vi "Ib.vi"(0 "Case":enum16{"100uA", "200uA", "300uA"}(ring), 1 "Zasilacz BM572":refnum<visa-resource-name>) -> (2 "COMMAND":string)   [LabVIEW 2023]
doc: "Podajemy prad bazy i ustawiamy napicie na zasilaczu zgodne z danym prdem"
uses:
  Open_device_2018.llb/Select_Instr.ctl
panel:
  out "result string":string
  out "ERROR\nERROR":errorcluster
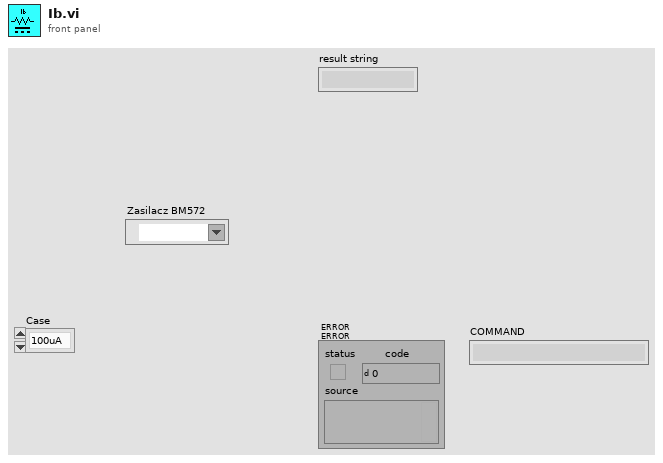
[diagram p1: front panel]
types:
  T1 = typedef "Select_Instr.ctl" = string
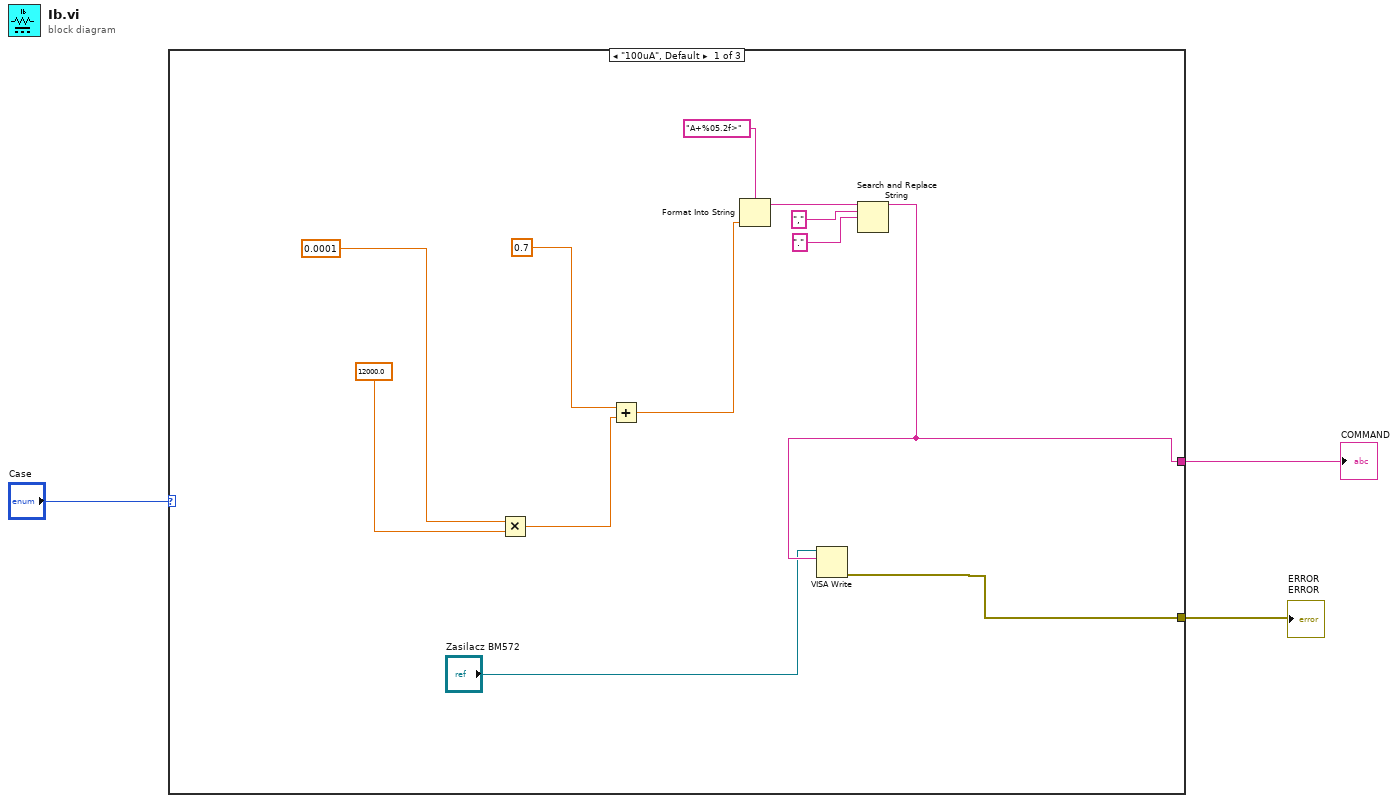
[diagram p0: block diagram]
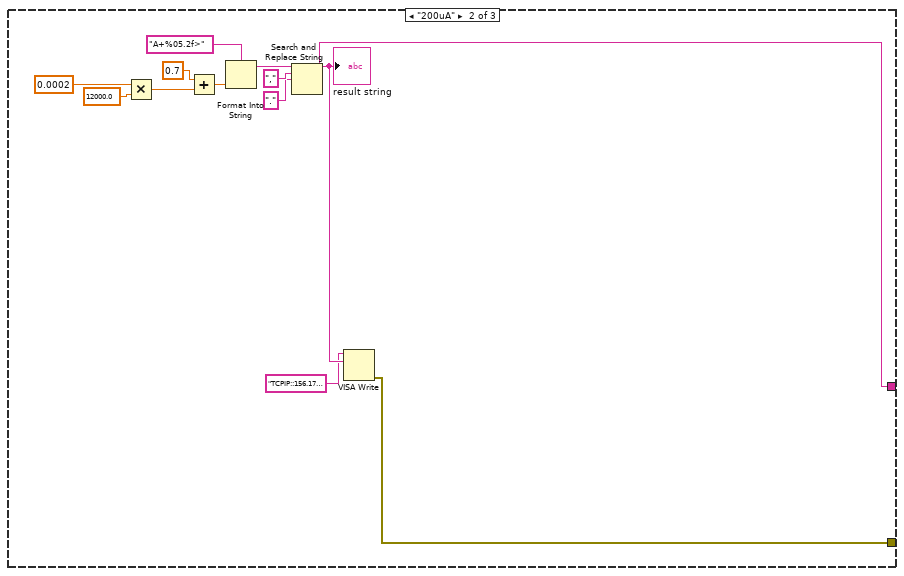
[diagram p2: hidden frame]
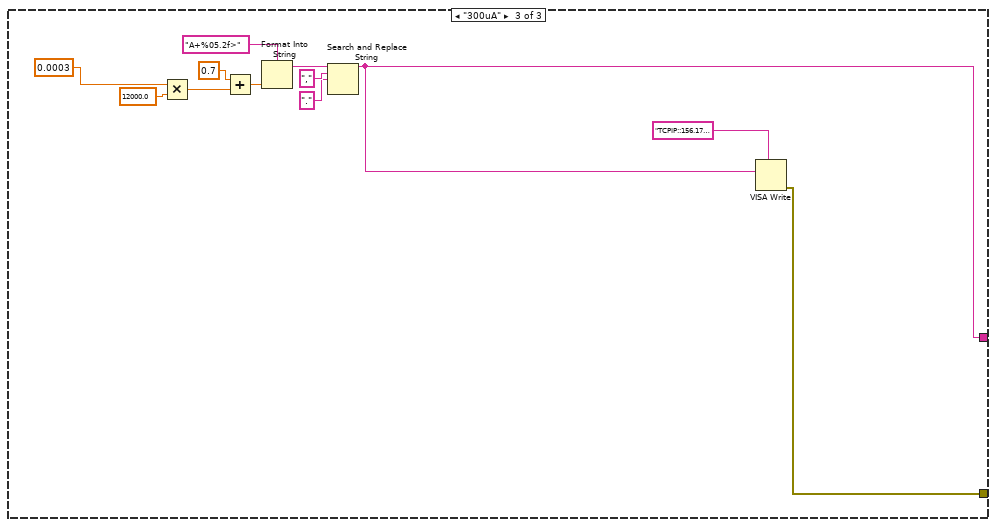
[diagram p3: hidden frame]
diagram:
  n1 = case shown="\"100uA\", Default" "Case" {
    tunnel: [w6 w18 w29] -> w3
    tunnel: [w7 w19 w31] -> w2
    frame "100uA", Default {
      n2 = Multiply(x=0.0001 ("Ib [A]"), y=12000.0) -> (x*y=w13:dbl)
      n3 = Add(x=0.7, y=w13) -> (x+y=w14:dbl)
      n4 = Format Into String(format string="A+%05.2f>" ("initial string"), w14) -> (resulting string=w15:string)  [unwired: 2 in, 1 out]
      n5 = Search and Replace String(input string=w15, search string=",", replace string="." ("replace string (\"\")")) -> (result string=w7:string)  [unwired: 5 in, 3 out]
      n6 = VISA Write(VISA resource name="Zasilacz BM572", write buffer=w7) -> (error out=w6:errorcluster)  [unwired: 1 in, 2 out]
    }
    frame "200uA" {
      n7 = Multiply(x=0.0002 ("Ib [A]"), y=12000.0) -> (x*y=w26:dbl)
      n8 = Add(x=0.7, y=w26) -> (x+y=w24:dbl)
      n9 = Format Into String(format string="A+%05.2f>" ("initial string"), w24) -> (resulting string=w22:string)  [unwired: 2 in, 1 out]
      n10 = Search and Replace String(input string=w22, search string=",", replace string="." ("replace string (\"\")")) -> (result string=w19:string)  [unwired: 5 in, 3 out]
      "result string" <- w19
      n11 = VISA Write(VISA resource name=T1 "TCPIP::156.17.45.35::inst18::INSTR" ("Select_Instrument"), write buffer=w19) -> (error out=w18:errorcluster)  [unwired: 1 in, 2 out]
    }
    frame "300uA" {
      n12 = Multiply(x=0.0003 ("Ib [A]"), y=12000.0) -> (x*y=w37:dbl)
      n13 = Add(x=0.7, y=w37) -> (x+y=w38:dbl)
      n14 = Format Into String(format string="A+%05.2f>" ("initial string"), w38) -> (resulting string=w39:string)  [unwired: 2 in, 1 out]
      n15 = Search and Replace String(input string=w39, search string=",", replace string="." ("replace string (\"\")")) -> (result string=w31:string)  [unwired: 5 in, 3 out]
      n16 = VISA Write(VISA resource name=T1 "TCPIP::156.17.45.35::inst18::INSTR" ("Select_Instrument"), write buffer=w31) -> (error out=w29:errorcluster)  [unwired: 1 in, 2 out]
    }
  }
  "ERROR\nERROR" <- w3
  "COMMAND" <- w2
